vi "Building_Origin_of_Subtrack_Merging_101-1.vi"(4 "[IN] Indexes \nfor Jumps":i32[](array[numeric]), 5 "error IN":errorcluster, 6 "[IN] Subtrack":T1, 8 "[IN] Still connected\ntracks in group":T2) -> (0 "error OUT":errorcluster, 1 "[OUT] Subtrack":T1, 2 "[OUT] Last point in subtrack":i32)   [LabVIEW 2013]
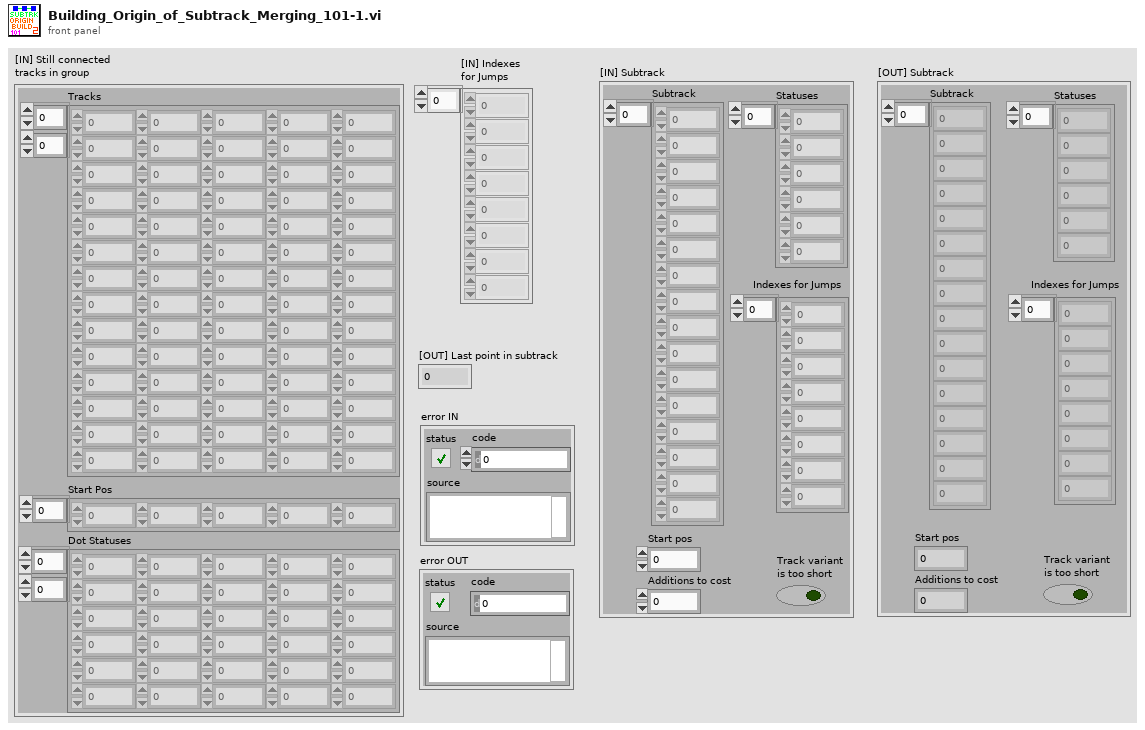
[diagram p1: front panel]
types:
  T1 = cluster{"Subtrack":dbl[], "Statuses":i16[], "Start pos":i32, "Additions to cost":i8, "Track variant \nis too short":bool, "Indexes for Jumps":i32[]}
  T2 = cluster{"Tracks":dbl[][], "Start Pos":i32[], "Dot Statuses":i16[][]}
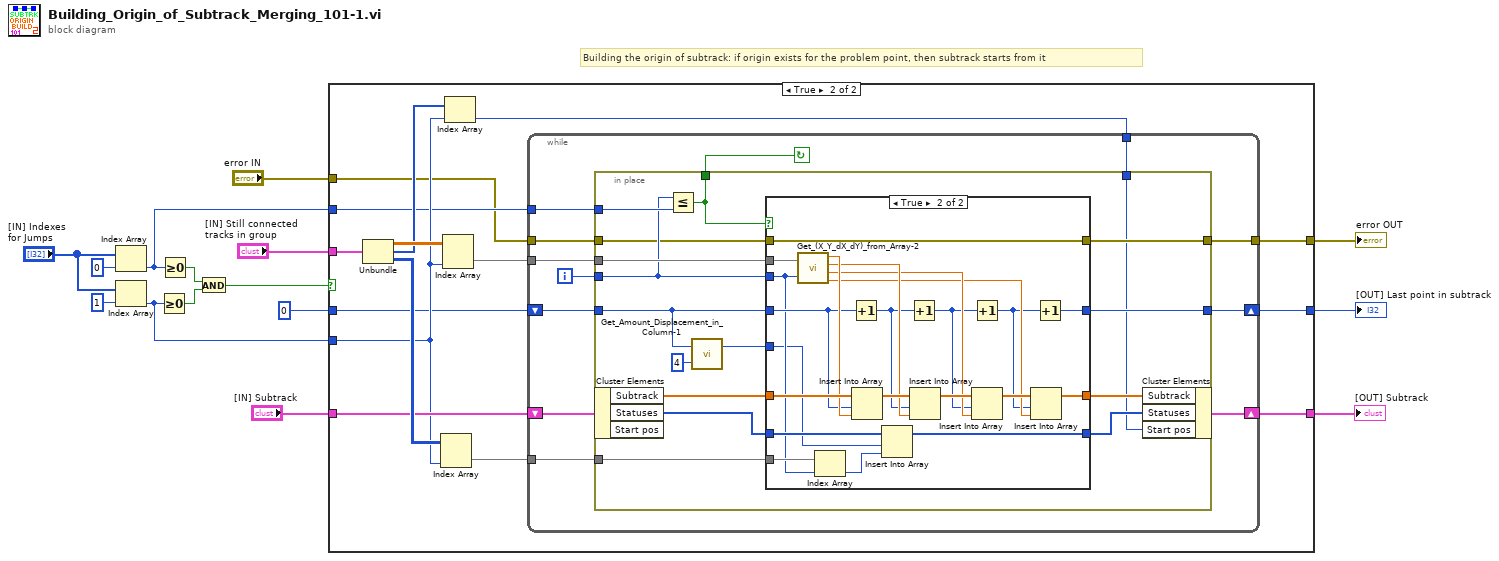
[diagram p0: block diagram]
diagram:
  # "Building the origin of subtrack: if origin exists for the problem point, then subtrack starts from it"
  n1 = Index Array(array="[IN] Indexes \nfor Jumps", index=0) -> (element=w4:i32)
  n2 = Index Array(array="[IN] Indexes \nfor Jumps", index=1) -> (element=w5:i32)
  n3 = Greater Or Equal To 0?(x=w5) -> (x >= 0?=w6:bool)
  n4 = Greater Or Equal To 0?(x=w4) -> (x >= 0?=w7:bool)
  n5 = And(x=w7, y=w6) -> (x .and. y?=w3:bool)
  n6 = case shown="True" w3 {
    tunnel: "[IN] Still connected\ntracks in group" -> [_ w33]
    tunnel: [w16 w26] -> w14
    tunnel: [w18 w25] -> w13
    tunnel: "[IN] Subtrack" -> [w17 w24]
    tunnel: [w17 w23] -> w8
    tunnel: w5 -> [_ w22]
    tunnel: w4 -> [_ w21]
    tunnel: "error IN" -> [w18 w20]
    tunnel: 0 -> [w16 w19]
    frame False {
    }
    frame True {
      n7 = Unbundle(w33) -> ("Tracks"=w32:dbl[][], "Start Pos"=w30:i32[], "Dot Statuses"=w28:i16[][])
      n8 = Index Array(array=w28, index (col)=w22) -> (element=w27:i16[])  [unwired: 1 in]
      n9 = Index Array(array=w32, index (col)=w22) -> (element=w31:dbl[])  [unwired: 1 in]
      n10 = Index Array(array=w30, index=w22) -> (element=w29:i32)
      n11 = while {
        tunnel: w31 -> [w45]
        tunnel: w27 -> [w43]
        shift-right: [w34] -> w23
        shift-left: w24 -> [w35]
        tunnel: w21 -> [w42]
        tunnel: w20 -> [w40]
        tunnel: [w39] -> w25
        tunnel: w29 -> [w38]
        shift-right: [w37] -> w26
        shift-left: w19 -> [w36]
        i -> [w41]
        stop <- w44 continue-if-true
        n12 = in-place {
          in-place-border: w45 -> [w61]
          in-place-border: [w60] -> w44
          in-place-border: w43 -> [w59]
          in-place-border: w42 -> [w58]
          in-place-border: w41 -> [w57]
          in-place-border: w40 -> [w56]
          in-place-border: [w55] -> w39
          in-place-border: w38 -> [w46]
          in-place-border: [w54] -> w37
          in-place-border: w36 -> [w52]
          n13 = in-place-cluster #1(w35) -> ("Subtrack"=w50:dbl[], "Statuses"=w49:i16[])  [unwired: 1 out]
          n14 = Less Or Equal?(x=w57, y=w58) -> (x <= y?=w60:bool)
          n15 = call "Get_Amount_Displacement_in_Column-1.vi"("multiplier"=4, "# Rows"=w52) -> ("Displ amount"=w51:i32)  [unwired: 1 out]
          n16 = case shown="True" w60 {
            tunnel: w61 -> [_ w87]
            tunnel: w50 -> [w64 w86]
            tunnel: w52 -> [w62 w84]
            tunnel: w57 -> [_ w73]
            tunnel: w49 -> [w65 w75]
            tunnel: w59 -> [_ w74]
            tunnel: [w64 w71] -> w48
            tunnel: [w65 w70] -> w47
            tunnel: w56 -> [w63 w69]
            tunnel: [w63 w69] -> w55
            tunnel: [w62 w66] -> w54
            tunnel: w51 -> [_ w68]
            frame False {
            }
            frame True {
              n17 = call "Get_(X_Y_dX_dY)_from_Array-2.vi"("(X,Y,dX,dY)"=w87, "Index of Displacement"=w73) -> ("X"=w85:dbl, "Y"=w82:dbl, "dX"=w79:dbl, "dY"=w76:dbl)
              n18 = Index Array(array=w74, index=w73) -> (element=w72:i16)
              n19 = Increment(x=w84) -> (x+1=w80:i32)
              n20 = Insert Into Array(array=w86, index=w84, new element=w85) -> (w83:dbl[])
              n21 = Insert Into Array(array=w75, index=w68, new element=w72) -> (w70:i16[])
              n22 = Increment(x=w80) -> (x+1=w78:i32)
              n23 = Insert Into Array(array=w83, index=w80, new element=w82) -> (w81:dbl[])
              n24 = Increment(x=w78) -> (x+1=w67:i32)
              n25 = Insert Into Array(array=w81, index=w78, new element=w79) -> (w77:dbl[])
              n26 = Insert Into Array(array=w77, index=w67, new element=w76) -> (w71:dbl[])
              n27 = Increment(x=w67) -> (x+1=w66:i32)
            }
          }
          n28 = in-place-cluster #1("Subtrack"=w48, "Statuses"=w47, "Start pos"=w46) -> (w34:T1)
        }
      }
    }
  }
  "[OUT] Last point in subtrack" <- w14
  "error OUT" <- w13
  "[OUT] Subtrack" <- w8
